vi "Convert dB Attenuation to Bits.vi"(4 "Attenuation Value (0 dB)":dbl min=0.0 max=63.75 step=0.25 format="%.2f") -> (1 "Binary VA Value":u32 format="%.0b")   [LabVIEW 2011]
doc: "Accepts the requested decimal attenuation value, and outputs an unsigned, 8-bit integer corresponding to the bits to be set on the Weinschel Model 5312 64 dB x 0.25 dB step attenuator.\n\nIf a requested value is out of range, the maximum or minimum attenutation setting is returned.\n\nThe output of this .vi is suitable for passing directly to the Write to Digital Port.vi in the standard NI toolbox."
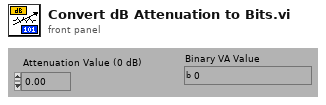
[diagram p1: front panel]
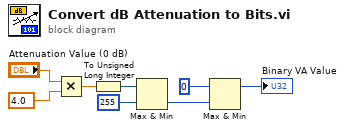
[diagram p0: block diagram]
diagram:
  n1 = Multiply(x="Attenuation Value (0 dB)", y=4.0) -> (x*y=w6:dbl)
  n2 = To Unsigned Long Integer(number=w6) -> (unsigned 32bit integer=w1:u32)
  n3 = Max & Min(x=w1, y=u32 255) -> (min(x,y)=w4:u32)  [unwired: 1 out]
  n4 = Max & Min(x=u32 0 ("y"), y=w4) -> (max(x,y)=→"Binary VA Value":u32)  [unwired: 1 out]
